vi "set_visa.vi"(8 "error in (no error)":errorcluster, 10 "visa array":refnum<visa-resource-name>[](array[refnum]), 11 "SignalWriterMH110203USBStepperMotor in":refnum<class "SignalWriterMH110203USBStepperMotor.lvclass">) -> (0 "error out":errorcluster, 3 "SignalWriterMH110203USBStepperMotor out":refnum<class "SignalWriterMH110203USBStepperMotor.lvclass">)   [LabVIEW 2010, in "SignalWriterMH110203USBStepperMotor.lvclass"]
uses:
  SignalWriterMH110203USBStepperMotor.lvclass
  SignalWriterMH110203USBStepperMotor.lvclass/SignalWriterMH110203USBStepperMotor.ctl
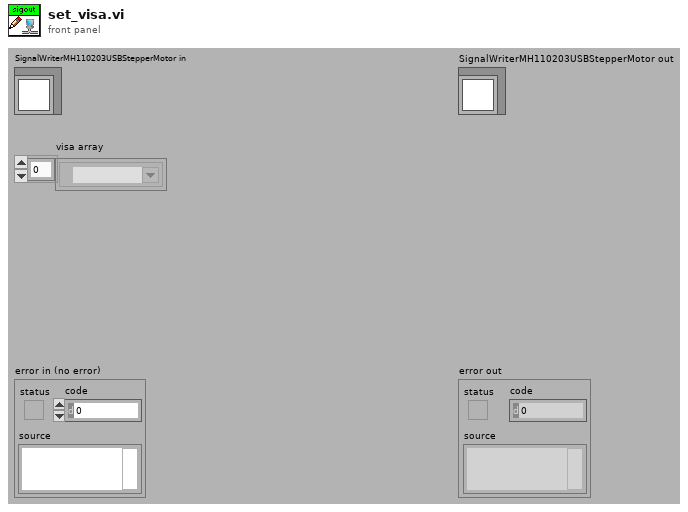
[diagram p1: front panel]
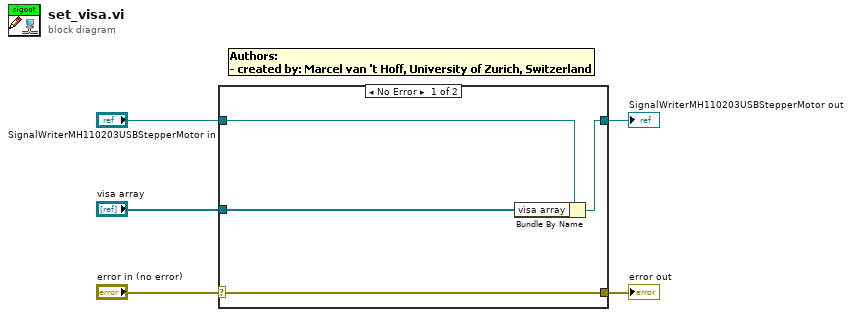
[diagram p0: block diagram]
diagram:
  n1 = case shown="No Error" "error in (no error)" {
    selector: "error in (no error)" -> [w9 w10]
    tunnel: [w9 w10] -> w4
    tunnel: [w7 w11] -> w2
    tunnel: "SignalWriterMH110203USBStepperMotor in" -> [w8 w11]
    tunnel: "visa array" -> [w6 _]
    frame No Error {
      n2 = Bundle By Name(cluster=w8, "visa array"=w6) -> (w7:refnum<class "SignalWriterMH110203USBStepperMotor.lvclass">)
    }
    frame Error {
    }
  }
  "error out" <- w4
  "SignalWriterMH110203USBStepperMotor out" <- w2
